vi "Adress test.vi"() -> ()   [LabVIEW 2017]
uses:
  <vilib>/Plasmionique/MB Master/MB_Master_Serial/MB_Master_Serial.lvclass
  D:/Program Files (x86)/National Instruments/LabVIEW 2017/vi.lib/Plasmionique/MB Master/MB_Master/MB_Master.lvclass
  <vilib>/Plasmionique/MB Master/MB Master.lvlib
panel:
  out "Registers":u16[](array[numeric])
  out "Error out":errorcluster
  out "code":i32
  in  "Slave ID":u8=2
  in  "VISA Resource":refnum<visa-resource-name>="COM8"
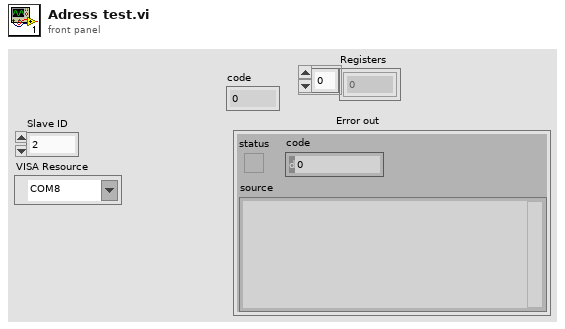
[diagram p1: front panel]
types:
  T1 = cluster{"baud rate (bps)":u32, "stop bits":u16, "parity":u16, "flow control":u16, "timeout":u32, "retries":i32}
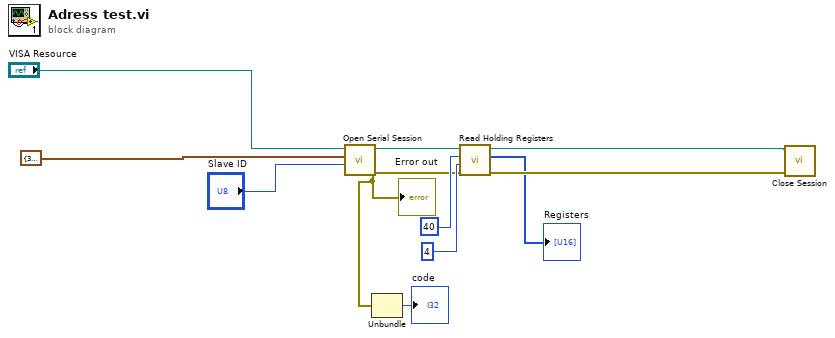
[diagram p0: block diagram]
diagram:
  n1 = call <vilib>:"Open Serial Session.vi"("Slave ID"="Slave ID", "Serial Config"=T1 {"baud rate (bps)"=38400, "stop bits"=10, "parity"=0, "flow control"=0, "timeout"=1000, "retries"=1}, "VISA Resource"="VISA Resource") -> ("Error out"=w4:errorcluster, "MB_Serial session"=w7:refnum<class "MB_Master_Serial.lvclass">)  [unwired: 7 in]
  "Error out" <- w4
  n2 = Unbundle(w4) -> ("code"=→"code":i32)  [unwired: 2 out]
  n3 = call <vilib>:"Read Holding Registers.vi"("error in (no error)"=w4, "quantity"=u16 4, "starting address"=u16 40, "MB session in"=w7) -> ("error out"=w2:errorcluster, "Registers"=→"Registers":u16[], "MB session out"=w3:refnum<class "MB_Master_Serial.lvclass">)  [unwired: 5 in]
  n4 = call-dynamic "Close Session.vi"("error in (no error)"=w2, "MB_Serial session"=w3) -> ()  [unwired: 9 in, 1 out]
